vi "NI_9210_Config.vi"(8 "error in":errorcluster, 11 "task in":refnum<k21>) -> (0 "error out":errorcluster, 3 "task out":refnum<k21>)   [LabVIEW 2022 SP3]
uses:
  <vilib>/DAQmx/create/channels.llb/DAQmx Create Channel (AI-Temperature-Thermocouple).vi
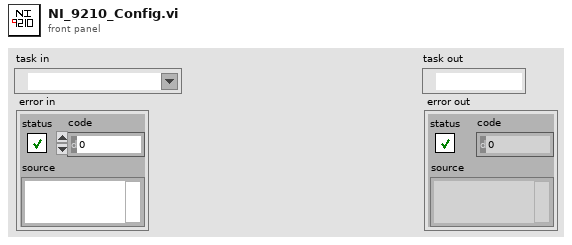
[diagram p1: front panel]
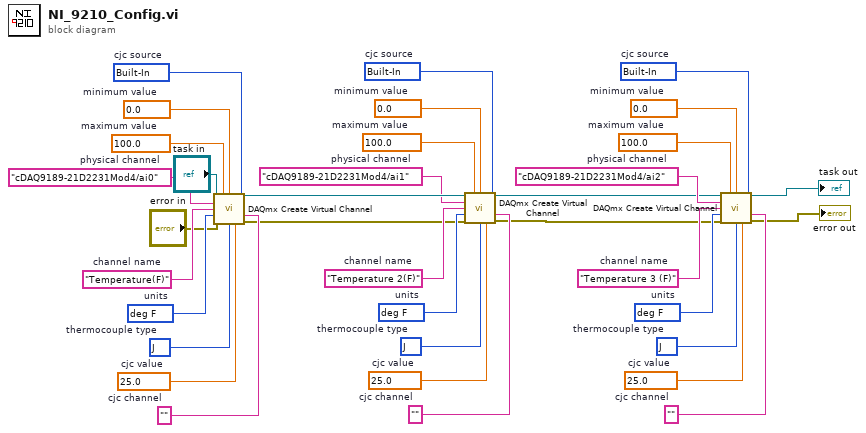
[diagram p0: block diagram]
diagram:
  w6 = 10200 items=["Built-In"=10200, "Constant Value"=10116, "Channel"=10113]  # cjc source
  w8 = ""  # cjc channel
  w9 = 25.0  # cjc value
  w10 = 10072 items=["J"=10072, "K"=10073, "N"=10077, "R"=10082, "S"=10085, "T"=10086, "B"=10047, "E"=10055]  # thermocouple type
  w11 = 10144 items=["deg C"=10143, "deg F"=10144, "Kelvins"=10325, "deg R"=10145, "From Custom Scale"=10065]  # units
  w7 = "Temperature 3 (F)"  # channel name
  w12 = 0.0  # minimum value
  w13 = 100.0  # maximum value
  w5 = "cDAQ9189-21D2231Mod4/ai2"  # physical channel
  w17 = 10200 items=["Built-In"=10200, "Constant Value"=10116, "Channel"=10113]  # cjc source
  w19 = ""  # cjc channel
  w20 = 25.0  # cjc value
  w21 = 10072 items=["J"=10072, "K"=10073, "N"=10077, "R"=10082, "S"=10085, "T"=10086, "B"=10047, "E"=10055]  # thermocouple type
  w22 = 10144 items=["deg C"=10143, "deg F"=10144, "Kelvins"=10325, "deg R"=10145, "From Custom Scale"=10065]  # units
  w18 = "Temperature 2(F)"  # channel name
  w23 = 0.0  # minimum value
  w24 = 100.0  # maximum value
  w14 = "cDAQ9189-21D2231Mod4/ai1"  # physical channel
  w27 = 10200 items=["Built-In"=10200, "Constant Value"=10116, "Channel"=10113]  # cjc source
  w29 = ""  # cjc channel
  w30 = 25.0  # cjc value
  w31 = 10072 items=["J"=10072, "K"=10073, "N"=10077, "R"=10082, "S"=10085, "T"=10086, "B"=10047, "E"=10055]  # thermocouple type
  w32 = 10144 items=["deg C"=10143, "deg F"=10144, "Kelvins"=10325, "deg R"=10145, "From Custom Scale"=10065]  # units
  w28 = "Temperature(F)"  # channel name
  w33 = 0.0  # minimum value
  w34 = 100.0  # maximum value
  w35 = "cDAQ9189-21D2231Mod4/ai0"  # physical channel
  n1 = call-poly <vilib>:"DAQmx Create Virtual Channel.vi"("task in"="task in", "maximum value"=w34, "minimum value"=w33, "physical channels"=w35, "cjc source"=w27, "name to assign"=w28, "units"=w32, "cjc channel"=w29, "error in"="error in", "thermocouple type"=w31, "cjc value"=w30) -> ("task out"=w16:refnum<k21>, "error out"=w15:errorcluster)  [unwired: 3 in]
  n2 = call-poly <vilib>:"DAQmx Create Virtual Channel.vi"("task in"=w16, "maximum value"=w24, "minimum value"=w23, "physical channels"=w14, "cjc source"=w17, "name to assign"=w18, "units"=w22, "cjc channel"=w19, "error in"=w15, "thermocouple type"=w21, "cjc value"=w20) -> ("task out"=w4:refnum<k21>, "error out"=w3:errorcluster)  [unwired: 3 in]
  n3 = call-poly <vilib>:"DAQmx Create Virtual Channel.vi"("task in"=w4, "maximum value"=w13, "minimum value"=w12, "physical channels"=w5, "cjc source"=w6, "name to assign"=w7, "units"=w11, "cjc channel"=w8, "error in"=w3, "thermocouple type"=w10, "cjc value"=w9) -> ("task out"=→"task out":refnum<k21>, "error out"=→"error out":errorcluster)  [unwired: 3 in]
